vi "Read Data.vi"(8 "error in (no error)":errorcluster, 11 "Tool Path in":refnum<class "Tool Path.lvclass">) -> (0 "error out":errorcluster, 2 "Path.lvclass":refnum<class "Path.lvclass">, 3 "Tool Path out":refnum<class "Tool Path.lvclass">)   [LabVIEW 2019, in "Tool Path.lvclass"]
uses:
  Tool Path.lvclass
  Parse/ParsePaths/Path.lvclass
  Tool Path.lvclass/Tool Path.ctl
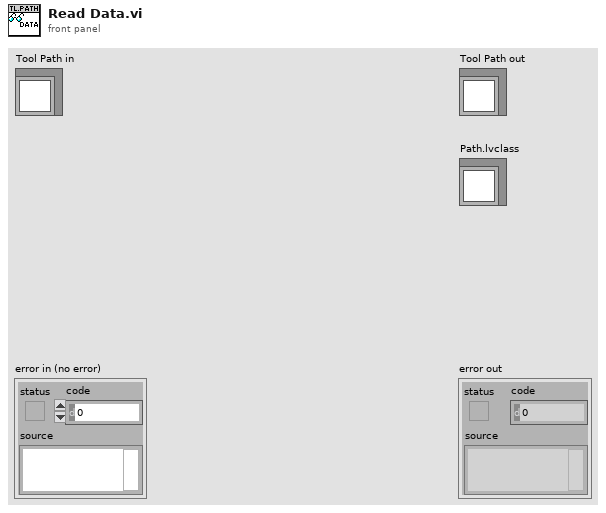
[diagram p1: front panel]
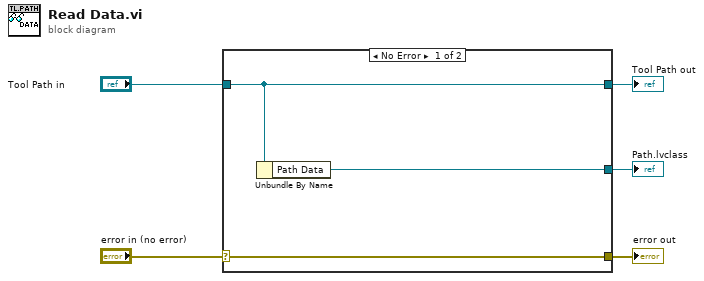
[diagram p0: block diagram]
diagram:
  n1 = case shown="No Error" "error in (no error)" {
    selector: "error in (no error)" -> [w8 w9]
    tunnel: [w8 w9] -> w4
    tunnel: [w7 w10] -> w2
    tunnel: "Tool Path in" -> [w7 w10]
    tunnel: [w6 _] -> w1
    frame No Error {
      n2 = Unbundle By Name(w7) -> ("Path Data"=w6:refnum<class "Path.lvclass">)
    }
    frame Error {
    }
  }
  "error out" <- w4
  "Tool Path out" <- w2
  "Path.lvclass" <- w1
